vi "Set Output Values.vi"(8 "error in (no error)":errorcluster, 11 "Spectrum Recorder in":refnum<class "Spectrum Recorder too.lvclass">) -> (0 "error out":errorcluster, 3 "Spectrum Recorder out":refnum<class "Spectrum Recorder too.lvclass">)   [LabVIEW 2016, in "Spectrum Recorder too.lvclass"]
uses:
  Spectrum Recorder too.lvclass
  Spectrum Recorder too.lvclass/Spectrum Recorder too.ctl
  Read Spectrum Recorder Configuration.vi
  Read RP transceiver.vi
  Write RP transceiver.vi
  NHMFL_Core/Libraries/Red Pitaya/RP Core/RP Transceiver/RP Transceiver.lvclass
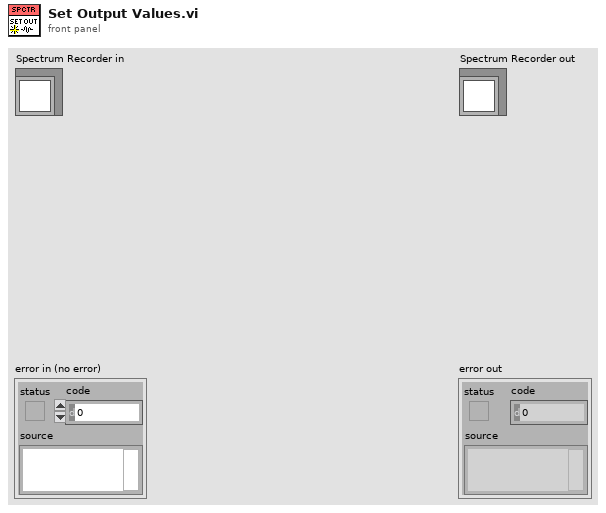
[diagram p1: front panel]
types:
  T1 = typedef "Spectrum Configuration.ctl" = cluster{"Start frequency":dbl, "End frequency":dbl, "Frequency step":dbl, "Step duration":dbl, "Red Pitaya address":string, "Open plot \non start":bool, "Focus region centers":dbl[], "Regions width":dbl, "Out-of-focus\nstep acceleration":i32}
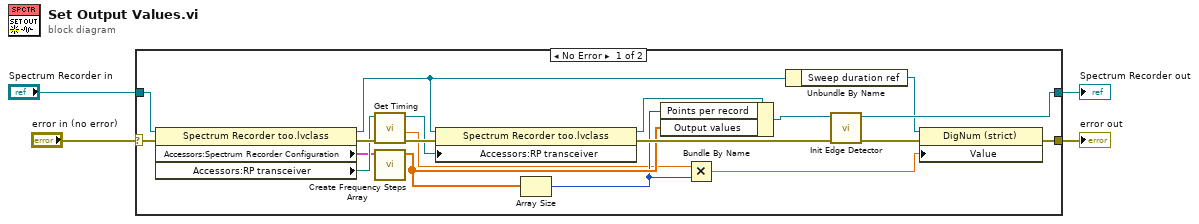
[diagram p0: block diagram]
diagram:
  n1 = case shown="No Error" "error in (no error)" {
    selector: "error in (no error)" -> [w19 w25]
    tunnel: [w8 w25] -> w3
    tunnel: [w14 w24] -> w1
    tunnel: "Spectrum Recorder in" -> [w21 w24]
    frame No Error {
      n2 = property class="Spectrum Recorder too.lvclass"(reference=w21, error in=w19) -> (reference out=w11:refnum<class "Spectrum Recorder too.lvclass">, error out=w20:errorcluster, "Accessors:Spectrum Recorder Configuration"=w13:T1, "Accessors:RP transceiver"=w18:refnum<class "RP Transceiver.lvclass">)
      n3 = call-dynamic "Get Timing.vi"("error in (no error)"=w20, "RP Transceiver in"=w18) -> ("error out"=w23:errorcluster, "dt"=w6:dbl, "RP Transceiver out"=w22:refnum<class "RP Transceiver.lvclass">)  [unwired: 5 in, 2 out]
      n4 = call "Create Frequency Steps Array.vi"("Spectrum Recorder Configuration"=w13) -> ("Steps"=w12:dbl[])  [unwired: 10 in]
      n5 = property class="Spectrum Recorder too.lvclass"(reference=w11, error in=w23, "Accessors:RP transceiver"=w22) -> (reference out=w17:refnum<class "Spectrum Recorder too.lvclass">, error out=w15:errorcluster)
      n6 = Array Size(array=w12) -> (size(s)=w7:i32)
      n7 = Bundle By Name(cluster=w17, "Points per record"=w7, "Output values"=w12) -> (w16:refnum<class "Spectrum Recorder too.lvclass">)
      n8 = Multiply(x=w6, y=w7) -> (x*y=w5:dbl)
      n9 = Unbundle By Name(w11) -> ("Sweep duration ref"=w10:refnum<vi>)
      n10 = call-dynamic "Init Edge Detector.vi"("error in (no error)"=w15, "Spectrum Recorder too in"=w16) -> ("error out"=w9:errorcluster, "Spectrum Recorder too out"=w14:refnum<class "Spectrum Recorder too.lvclass">)  [unwired: 8 in]
      n11 = property class="DigNum (strict)"(reference=w10, error in=w9, "Value"=w5) -> (error out=w8:errorcluster)  [unwired: 1 out]
    }
    frame Error {
    }
  }
  "error out" <- w3
  "Spectrum Recorder out" <- w1
